vi "weight_experimental.vi"(11 "PV weight":dbl caption="g" format="%#.0f") -> (1 "Q3":dbl caption="mg/s" format="%#.0f", 2 "Q 1":dbl caption="mg/s" format="%#.0f", 3 "Weight 1":dbl caption="g" format="%#.0f", 5 "This VI":refnum<vi>)   [LabVIEW 2019]
panel:
  in  "Tab Control":T1(tab)
  out "dM 3":dbl caption="g" format="%#.0f"
  out "dM 1":dbl caption="g" format="%#.0f"
  in  "Tare":dbl caption="g" format="%#.0f"
  in  "<0>":bool
  in  "<вес>":bool
  in  "k":dbl=1.0 caption="g" format="%#.3f"
  in  "Вес":dbl caption="g" format="%#.0f"
  # "Усреднение за 1 мин"
  # "(расход)"
  # "Усреднение за 3 мин"
  # "(расход)"
  # "Вес тары\n(полностью очистить бункер от продукта\nи запомнить PV weight или ввести вручную)."
  # "Вес тары\n(ввести фактический вес без учета тары\nили ввести k вручную)"
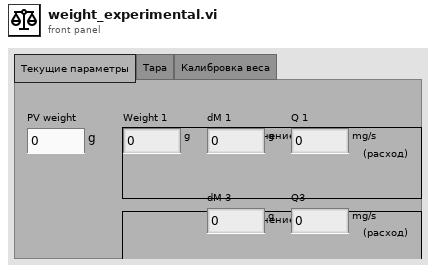
[diagram p1: front panel]
types:
  T1 = enum32{"Текущие параметры", "Тара", "Калибровка веса"}
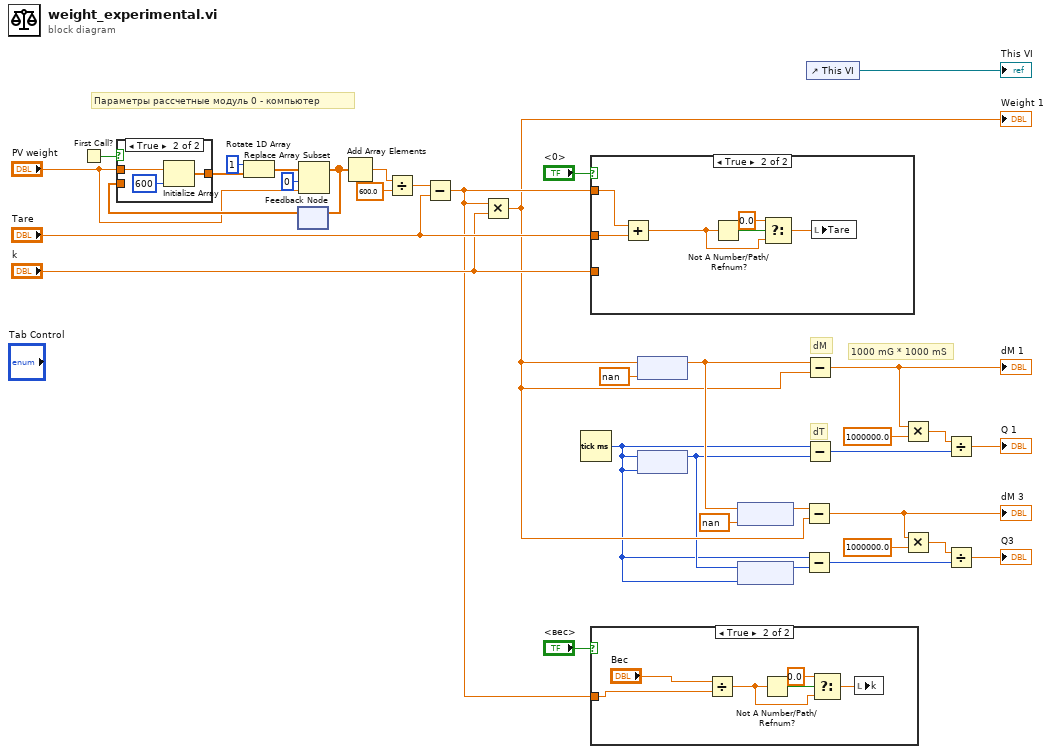
[diagram p0: block diagram]
diagram:
  # "1000 mG * 1000 mS"
  # "dM"
  # "dT"
  # "Параметры рассчетные модуль 0 - компьютер"
  n1 = First Call?() -> (First Call?: T/F=w28:bool)
  n2 = feedback #1() -> (w30:dbl[])  [unwired: 1 in]
  n3 = case shown="True" w28 {
    tunnel: [w36 w38] -> w29
    tunnel: "PV weight" -> [_ w37]
    tunnel: w30 -> [w36 _]
    frame False {
    }
    frame True {
      n4 = Initialize Array(w37, 600 ("dimension size")) -> (w38:dbl[])
    }
  }
  n5 = Rotate 1D Array(1:w29, 2:1 ("n")) -> (0:w34:dbl[])
  n6 = Replace Array Subset(array=w34, new element="PV weight", index=0) -> (w13:dbl[])
  n7 = feedback-in #1(w13) -> ()
  n8 = Add Array Elements(numeric array=w13) -> (sum=w31:dbl)
  n9 = Divide(x=w31, y=600.0) -> (x/y=w12:dbl)
  n10 = Subtract(x=w12, y="Tare") -> (x-y=w14:dbl)
  n11 = Multiply(x=w14, y="k") -> (x*y=w10:dbl)
  "Weight 1" <- w10
  n12 = Tick Count (ms)() -> (millisecond timer value=w6:u32)
  n13 = case shown="True" "<0>" {
    tunnel: "Tare" -> [_ w42]
    tunnel: w14 -> [_ w41]
    tunnel: "k" -> [_ _]
    frame False {
    }
    frame True {
      n14 = Add(x=w41, y=w42) -> (x+y=w40:dbl)
      n15 = Not A Number/Path/Refnum?(number/path/refnum=w40) -> (NaN/Path/Refnum?=w45:bool)
      n16 = Select(t=0.0 ("y"), s=w45, f=w40) -> (s? t:f=w43:dbl)
      n17 = local write "Tare"(w43) -> ()
    }
  }
  n18 = case shown="True" "<вес>" {
    tunnel: w14 -> [_ w46]
    frame False {
    }
    frame True {
      n19 = Divide(x="Вес", y=w46) -> (x/y=w49:dbl)
      n20 = Not A Number/Path/Refnum?(number/path/refnum=w49) -> (NaN/Path/Refnum?=w51:bool)
      n21 = Select(t=0.0 ("y"), s=w51, f=w49) -> (s? t:f=w48:dbl)
      n22 = local write "k"(w48) -> ()
    }
  }
  n23 = feedback #2(nan) -> (w23:dbl)
  n24 = feedback-in #2(w10) -> ()
  n25 = feedback #3(w6) -> (w8:u32)
  n26 = feedback-in #3(w6) -> ()
  n27 = feedback #4(nan) -> (w24:dbl)
  n28 = feedback-in #4(w23) -> ()
  n29 = feedback #5(w6) -> (w7:u32)
  n30 = feedback-in #5(w8) -> ()
  n31 = Subtract(x=w24, y=w10) -> (x-y=w2:dbl)
  "dM 3" <- w2
  n32 = Subtract(x=w6, y=w7) -> (x-y=w3:u32)
  n33 = Subtract(x=w23, y=w10) -> (x-y=w18:dbl)
  "dM 1" <- w18
  n34 = Subtract(x=w6, y=w8) -> (x-y=w16:u32)
  n35 = control-ref of="This VI"() -> (→"This VI":refnum<vi>)
  n36 = Multiply(x=w18, y=1000000.0) -> (x*y=w17:dbl)
  n37 = Multiply(x=w2, y=1000000.0) -> (x*y=w5:dbl)
  n38 = Divide(x=w17, y=w16) -> (x/y=→"Q 1":dbl)
  n39 = Divide(x=w5, y=w3) -> (x/y=→"Q3":dbl)
